vi "AutoAdjustYAlxesPosition.vi"(10 "YaxleNum":i32, 11 "XYGraph输入":refnum<vi>) -> (3 "显示的Y轴数":i32)   [LabVIEW 2015]
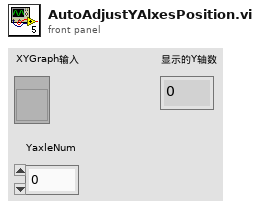
[diagram p1: front panel]
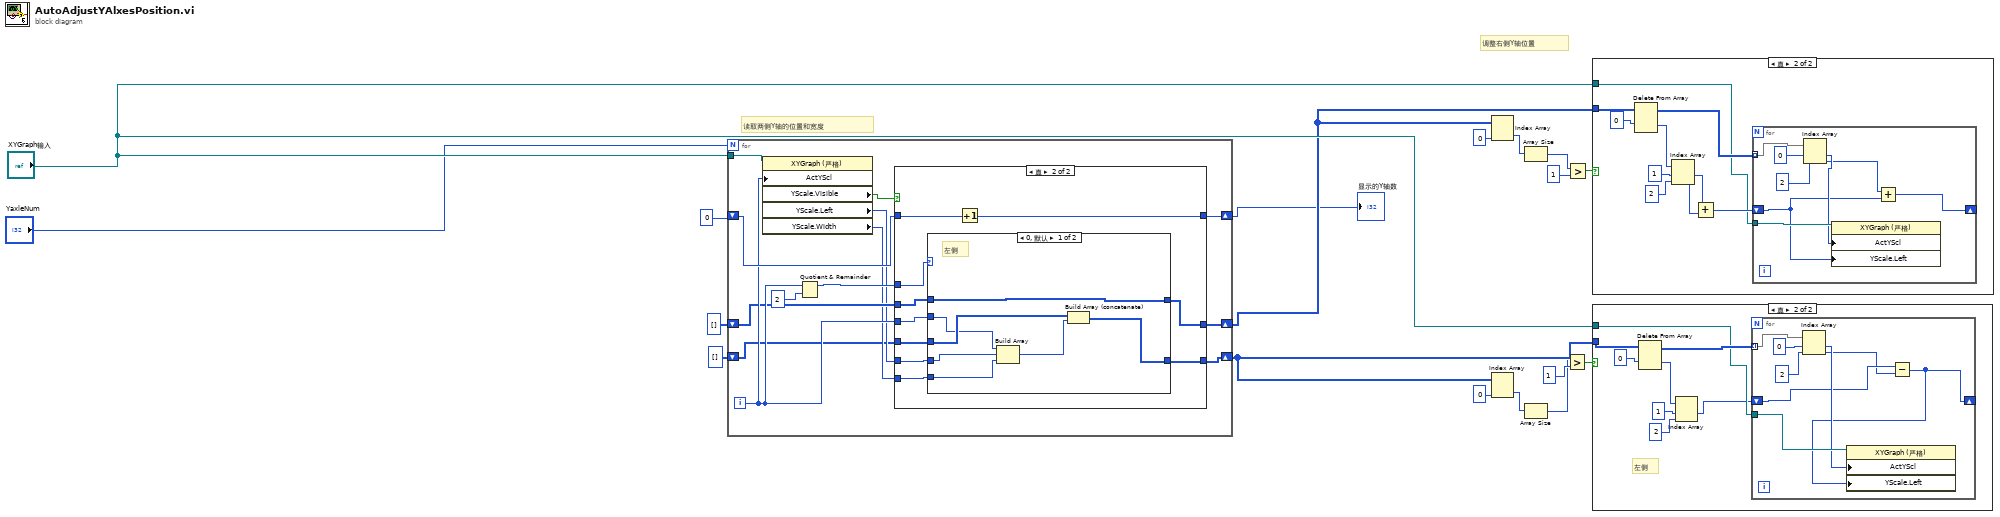
[diagram p0: block diagram]
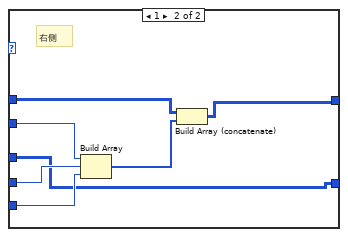
[diagram p5: hidden frame]
diagram:
  # "调整右侧Y轴位置"
  # "读取两侧Y轴的位置和宽度"
  n1 = for {
    N: "YaxleNum" -> [_]
    tunnel: "XYGraph输入" -> [w31]
    shift-right: [w28] -> w2
    shift-left: 0 -> [w29]
    shift-right: [w24] -> w17
    shift-left: u32[][] [] -> [w23]
    shift-right: [w19] -> w11
    shift-left: u32[][] [] -> [w20]
    i -> [w25]
    n2 = property class="XYGraph (严格)"(reference=w31, "ActYScl"=w25) -> ("YScale.Visible"=w30:bool, "YScale.Left"=w22:i32, "YScale.Width"=w21:u32)  [unwired: 1 in, 2 out]
    n3 = Quotient & Remainder(x=w25, y=2) -> (x-y*floor(x/y)=w26:i32)  [unwired: 1 out]
    n4 = case shown="真" w30 {
      tunnel: w29 -> [w34 w44]
      tunnel: [w34 w43] -> w28
      tunnel: w26 -> [_ w42]
      tunnel: w25 -> [_ w41]
      tunnel: [w33 w40] -> w24
      tunnel: w23 -> [w33 w39]
      tunnel: w22 -> [_ w38]
      tunnel: w21 -> [_ w37]
      tunnel: w20 -> [w32 w36]
      tunnel: [w32 w35] -> w19
      frame False {
      }
      frame True {
        n5 = case shown="0, 默认" w42 {
          tunnel: w41 -> [w47 w58]
          tunnel: [w51 w55] -> w40
          tunnel: w39 -> [w51 w53]
          tunnel: w38 -> [w46 w57]
          tunnel: w37 -> [w45 w56]
          tunnel: w36 -> [w49 w52]
          tunnel: [w48 w52] -> w35
          frame 0, Default {
            # "左侧"
            n6 = Build Array(w47, w46, w45) -> (w50:u32[])
            n7 = Build Array (concatenate)(w49, w50) -> (w48:u32[][])
          }
          frame 1 {
            # "右侧"
            n8 = Build Array(w58, w57, w56) -> (w54:u32[])
            n9 = Build Array (concatenate)(w53, w54) -> (w55:u32[][])
          }
        }
        n10 = Increment(x=w44) -> (x+1=w43:i32)
      }
    }
  }
  "显示的Y轴数" <- w2
  n11 = Index Array(array=w17, index (col)=0 ("禁用的索引 (列)")) -> (element=w16:u32[])  [unwired: 1 in]
  n12 = Index Array(array=w11, index (col)=0 ("禁用的索引 (列)")) -> (element=w10:u32[])  [unwired: 1 in]
  n13 = Array Size(array=w16) -> (size(s)=w13:i32)
  n14 = Array Size(array=w10) -> (size(s)=w7:i32)
  n15 = Greater?(x=w7, y=1) -> (0:w9:bool)
  n16 = Greater?(x=w13, y=1) -> (0:w15:bool)
  n17 = case shown="真" w9 {
    tunnel: w11 -> [_ w66]
    tunnel: "XYGraph输入" -> [_ w60]
    frame False {
    }
    frame True {
      # "左侧"
      n18 = Delete From Array(array=w66, index (row)=0 ("长度")) -> (deleted portion=w64:u32[], array with subset deleted=w61:u32[][])  [unwired: 2 in]
      n19 = Index Array(array=w64, index #1=1 ("索引"), index #2=2 ("索引")) -> (element #1=w59:u32)  [unwired: 1 out]
      n20 = for {
        tunnel: w61 -> [w73] mode=indexing
        shift-right: [w67] -> _
        shift-left: w59 -> [w69]
        tunnel: w60 -> [w74]
        n21 = Index Array(array=w73, index #1=0 ("索引"), index #2=2 ("索引")) -> (element #1=w70:u32, element #2=w68:u32)
        n22 = Subtract(x=w69, y=w68) -> (x-y=w67:u32)
        n23 = property class="XYGraph (严格)"(reference=w74, "ActYScl"=w70, "YScale.Left"=w67) -> ()  [unwired: 1 in, 2 out]
      }
    }
  }
  n24 = case shown="真" w15 {
    tunnel: w17 -> [_ w84]
    tunnel: "XYGraph输入" -> [_ w75]
    frame False {
    }
    frame True {
      n25 = Delete From Array(array=w84, index (row)=0 ("长度")) -> (deleted portion=w82:u32[], array with subset deleted=w79:u32[][])  [unwired: 2 in]
      n26 = Index Array(array=w82, index #1=1 ("索引"), index #2=2 ("索引")) -> (element #1=w78:u32, element #2=w77:u32)
      n27 = Add(x=w78, y=w77) -> (x+y=w76:u32)
      n28 = for {
        tunnel: w79 -> [w91] mode=indexing
        shift-right: [w85] -> _
        shift-left: w76 -> [w87]
        tunnel: w75 -> [w92]
        n29 = Index Array(array=w91, index #1=0 ("索引"), index #2=2 ("索引")) -> (element #1=w88:u32, element #2=w86:u32)
        n30 = property class="XYGraph (严格)"(reference=w92, "ActYScl"=w88, "YScale.Left"=w87) -> ()  [unwired: 1 in, 2 out]
        n31 = Add(x=w86, y=w87) -> (x+y=w85:u32)
      }
    }
  }
